vi "RemoveClassNameFromMethod.vi"(1 "MethodVINameIn":string, 3 "ClassName":string) -> (15 "MethodVINameOut":string)   [LabVIEW 2016, in "ClassReader.lvclass"]
uses:
  <resource>/Framework/Providers/Open_GDS/ClassProviders/Provider_BaseClassInterface/ClassReader_class/ClassReader.lvclass
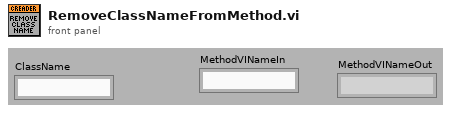
[diagram p1: front panel]
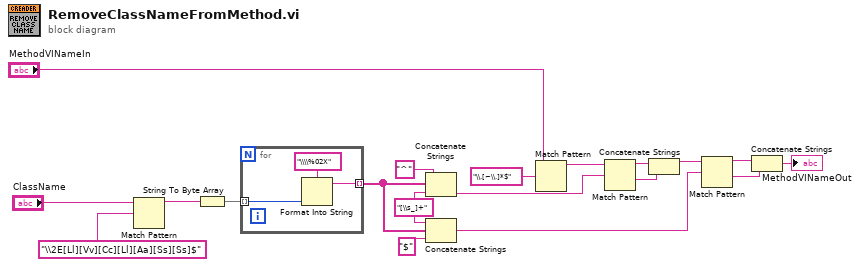
[diagram p0: block diagram]
diagram:
  w4 = "[\\s_]+" ("string")
  n1 = Match Pattern(string="ClassName", regular expression="\\2E[Ll][Vv][Cc][Ll][Aa][Ss][Ss]$") -> (before substring=w8:string)  [unwired: 1 in, 3 out]
  n2 = String To Byte Array(string=w8) -> (unsigned byte array=w7:u8[])
  n3 = for {
    tunnel: w7 -> [w22] mode=indexing
    tunnel: [w20] -> w6 mode=indexing
    n4 = Format Into String(format string="\\\\%02X", w22) -> (resulting string=w20:string)  [unwired: 2 in, 1 out]
  }
  n5 = Concatenate Strings("^", w6, w4) -> (w16:string)
  n6 = Concatenate Strings(w4, w6, "$") -> (w17:string)
  n7 = Match Pattern(string="MethodVINameIn", regular expression="\\.[~\\.]*$") -> (before substring=w14:string)  [unwired: 1 in, 3 out]
  n8 = Match Pattern(string=w14, regular expression=w16) -> (before substring=w13:string, after substring=w12:string)  [unwired: 1 in, 2 out]
  n9 = Concatenate Strings(w13, w12) -> (w11:string)
  n10 = Match Pattern(string=w11, regular expression=w17) -> (before substring=w10:string, after substring=w9:string)  [unwired: 1 in, 2 out]
  n11 = Concatenate Strings(w10, w9) -> (→"MethodVINameOut":string)
